vi "Test.vi"() -> ()   [LabVIEW 2014]
doc: "This VI is called when test mode begins, and will automatically be terminated when it ends. You can add manual or automatic tests and invoke them from the dashboard."
uses:
  <vilib>/Rock Robotics/WPI/Joystick/WPI_JoystickDeviceEnum.ctl
panel:
  out "Button 14":bool
  out "Button 13":bool
  out "Button 12":bool
  out "Button 11":bool
  out "Button 10":bool
  out "Analog 10":dbl
  out "Analog 9":dbl
  out "Analog 8":dbl
  out "Analog 7":dbl
  out "Analog 6":dbl
  out "Analog 5":dbl
  out "Analog 4":dbl
  out "Analog 3":dbl
  out "Analog 2":dbl
  out "Analog 1":dbl
  out "Analog 0":dbl
  out "Button 9":bool
  out "Button 8":bool
  out "Button 7":bool
  out "Button 6":bool
  out "Button 5":bool
  out "Button 4":bool
  out "Button 3":bool
  out "Button 2":bool
  out "Button 1":bool
  out "Button 0":bool
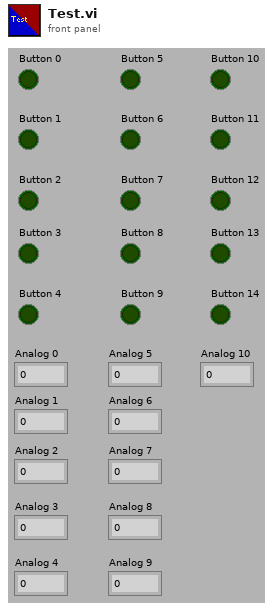
[diagram p1: front panel]
types:
  T1 = typedef "WPI_JoystickDeviceEnum.ctl" = enum16{"USB 0", "USB 1", "USB 2", "USB 3", "USB 4", "USB 5"}
  T2 = typedef "WPI_JoystickDevRef.ctl" = cluster{"Device":T1}
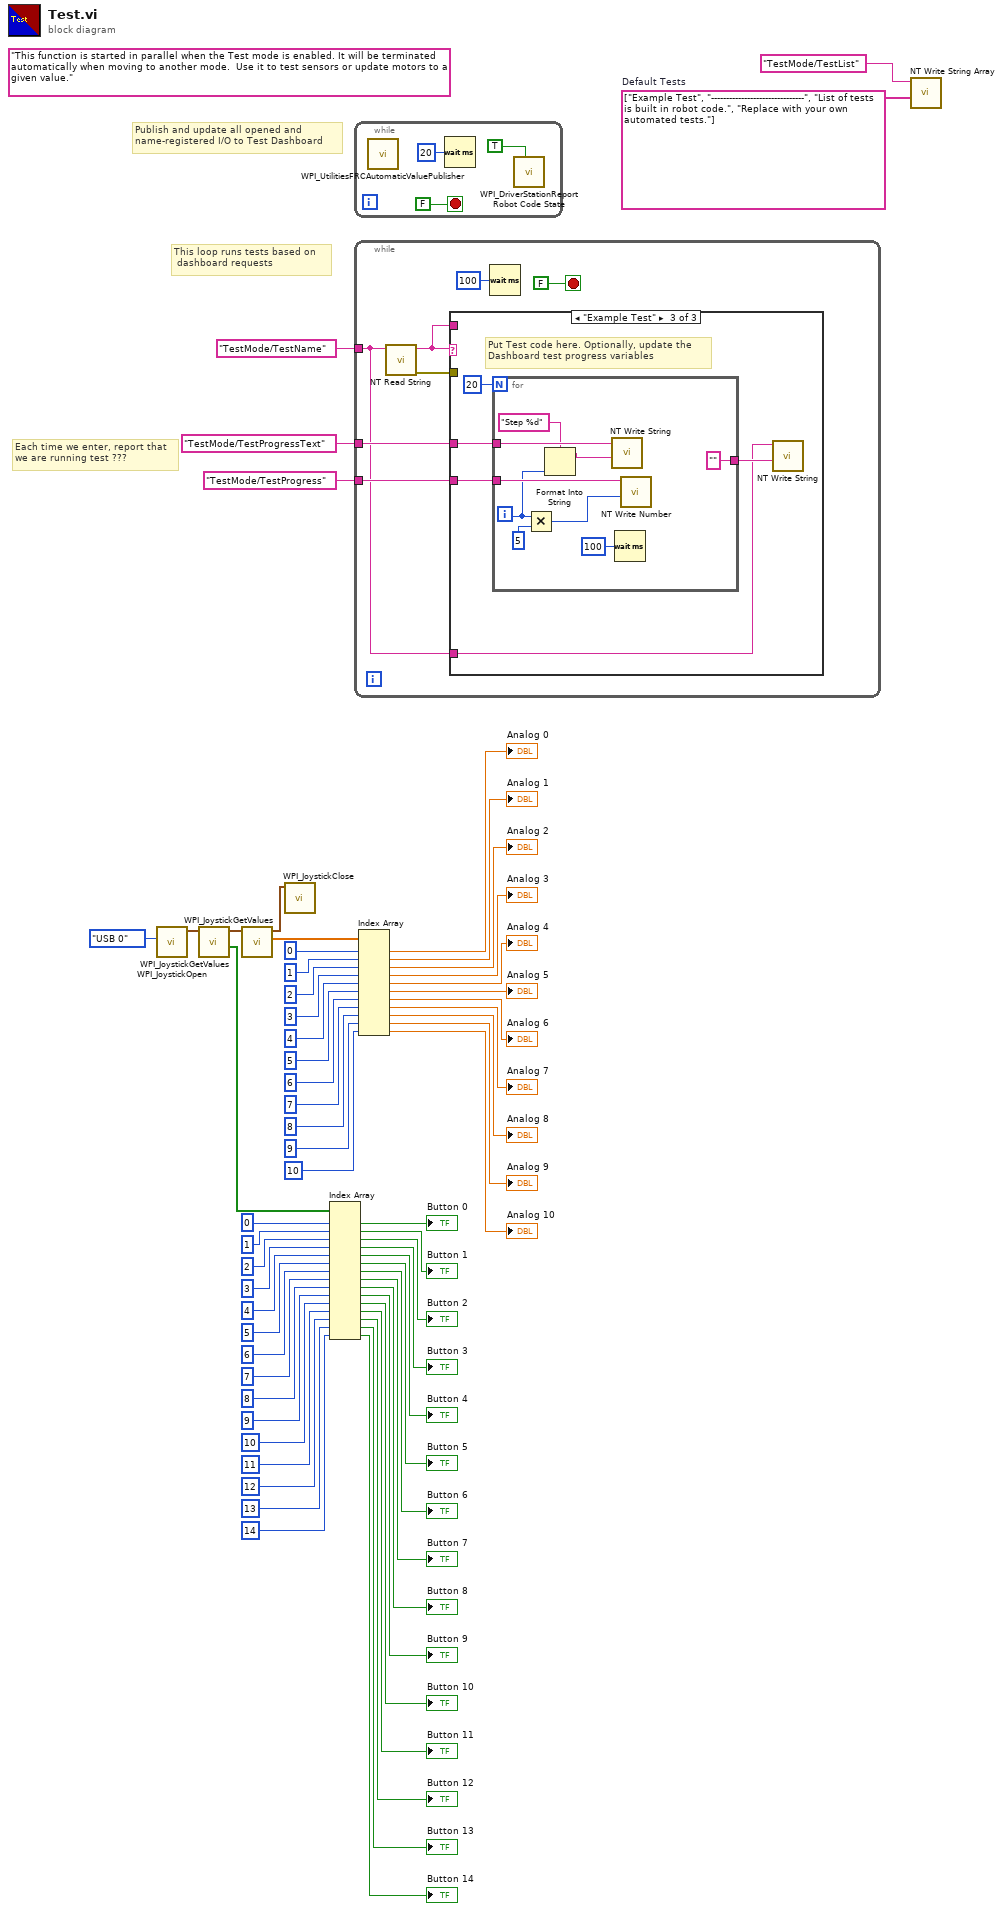
[diagram p0: block diagram]
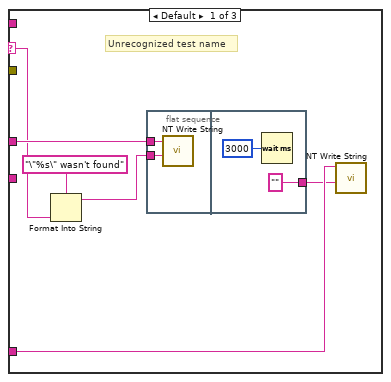
[diagram p2: hidden frame]
diagram:
  w60 = string[] ["Example Test", "-------------------------------", "List of tests is built in robot code.", "Replace with your own automated tests."]  # Default Tests
  (unwired) "This function is started in parallel when the Test mode is enabled. It will be terminated automatically when moving to another mode.  Use it to test sensors or update motors to a given value."
  # "This loop runs tests based on \n dashboard requests"
  # "Publish and update all opened and\nname-registered I/O to Test Dashboard"
  # "Each time we enter, report that\nwe are running test ???"
  n1 = call <vilib>:"WPI_JoystickOpen.vi"("JoystickDevice"=WPI_JoystickDeviceEnum."USB 0") -> ("JoystickDevRef"=w21:T2)  [unwired: 10 in]
  n2 = call <vilib>:"WPI_JoystickGetValues.vi"("JoystickDevRef"=w21) -> ("Buttons"=w51:bool[], "JoystickDevRef"=w22:T2)  [unwired: 6 in, 3 out]
  n3 = call <vilib>:"WPI_JoystickGetValues.vi"("JoystickDevRef"=w22) -> ("Axes"=w36:dbl[], "JoystickDevRef"=w23:T2)  [unwired: 6 in, 3 out]
  n4 = call <vilib>:"WPI_JoystickClose.vi"("JoystickDevRef"=w23) -> ()  [unwired: 11 in]
  n5 = Index Array(array=w51, index #1=0, index #2=1, index #3=2, index #4=3, index #5=4, index #6=5, index #7=6, index #8=7, index #9=8, index #10=9, index #11=10, index #12=11, index #13=12, index #14=13, index #15=14) -> (element #1=→"Button 0":bool, element #2=→"Button 1":bool, element #3=→"Button 2":bool, element #4=→"Button 3":bool, element #5=→"Button 4":bool, element #6=→"Button 5":bool, element #7=→"Button 6":bool, element #8=→"Button 7":bool, element #9=→"Button 8":bool, element #10=→"Button 9":bool, element #11=→"Button 10":bool, element #12=→"Button 11":bool, element #13=→"Button 12":bool, element #14=→"Button 13":bool, element #15=→"Button 14":bool)
  n6 = while {
    stop <- FALSE stop-if-true
    n7 = call <vilib>:"WPI_UtilitiesFRCAutomaticValuePublisher.vi"() -> ()  [unwired: 12 in]
    n8 = Wait (ms)(milliseconds to wait=u32 20) -> ()  [unwired: 1 out]
    n9 = call <vilib>:"WPI_DriverStationReport Robot Code State.vi"("Test"=TRUE ("Autonomous")) -> ()  [unwired: 10 in, 1 out]
  }
  n10 = while {
    tunnel: "TestMode/TestName" ("Name") -> [w68]
    tunnel: "TestMode/TestProgressText" ("Name") -> [w71]
    tunnel: "TestMode/TestProgress" ("Name") -> [w70]
    stop <- FALSE stop-if-true
    n11 = call <vilib>:"NT Read String.vi"("Name"=w68) -> ("error out"=w67:errorcluster, "String"=w69:string)  [unwired: 9 in]
    n12 = case shown="\"Example Test\"" w69 {
      selector: w69 -> [w78 _ _]
      tunnel: w68 -> [w75 _ w84]
      tunnel: w71 -> [w79 _ w87]
      tunnel: w70 -> [_ _ w88]
      tunnel: w69 -> [_ _ _]
      tunnel: w67 -> [_ _ _]
      frame Default {
        # "Unrecognized test name"
        n13 = Format Into String(format string="\"%s\" wasn't found" ("Name"), w78) -> (resulting string=w77:string)  [unwired: 2 in, 1 out]
        n14 = flat-sequence {
          tunnel: w79 -> [w80]
          tunnel: w77 -> [w81]
          tunnel: ["" ("Name")] -> w74
          frame #0 {
            n15 = call <vilib>:"NT Write String.vi"("String"=w81, "Name"=w80) -> ()  [unwired: 9 in, 1 out]
          }
          frame #1 {
            n16 = Wait (ms)(milliseconds to wait=u32 3000) -> ()  [unwired: 1 out]
          }
        }
        n17 = call <vilib>:"NT Write String.vi"("String"=w74, "Name"=w75) -> ()  [unwired: 9 in, 1 out]
      }
      frame "" {
        # "No test to run"
      }
      frame "Example Test" {
        # "Put Test code here. Optionally, update the\nDashboard test progress variables"
        n18 = for {
          N: 20 -> [_]
          tunnel: w88 -> [w97]
          tunnel: w87 -> [w95]
          tunnel: ["" ("String")] -> w85
          i -> [w92]
          n19 = Multiply(x=w92, y=u32 5 ("milliseconds to wait")) -> (x*y=w93:u32)
          n20 = Format Into String(format string="Step %d", w92) -> (resulting string=w90:string)  [unwired: 2 in, 1 out]
          n21 = call <vilib>:"NT Write String.vi"("String"=w90, "Name"=w95) -> ()  [unwired: 9 in, 1 out]
          n22 = Wait (ms)(milliseconds to wait=u32 100) -> ()  [unwired: 1 out]
          n23 = call <vilib>:"NT Write Number.vi"("Numeric"=w93, "Name"=w97) -> ()  [unwired: 9 in, 1 out]
        }
        n24 = call <vilib>:"NT Write String.vi"("String"=w85, "Name"=w84) -> ()  [unwired: 9 in, 1 out]
      }
    }
    n25 = Wait (ms)(milliseconds to wait=u32 100) -> ()  [unwired: 1 out]
  }
  n26 = Index Array(array=w36, index #1=0, index #2=1, index #3=2, index #4=3, index #5=4, index #6=5, index #7=6, index #8=7, index #9=8, index #10=9, index #11=10) -> (element #1=→"Analog 0":dbl, element #2=→"Analog 1":dbl, element #3=→"Analog 2":dbl, element #4=→"Analog 3":dbl, element #5=→"Analog 4":dbl, element #6=→"Analog 5":dbl, element #7=→"Analog 6":dbl, element #8=→"Analog 7":dbl, element #9=→"Analog 8":dbl, element #10=→"Analog 9":dbl, element #11=→"Analog 10":dbl)
  n27 = call <vilib>:"NT Write String Array.vi"("String Array"=w60, "Name"="TestMode/TestList") -> ()  [unwired: 9 in, 1 out]
